vi "ex14-7(withSubVI).vi"() -> ()   [LabVIEW 2014]
panel:
  out "·¸¦ì?65536(­¼ªk)":bool
  out "溢位?65536(除法)":bool
  in  "X":dbl
  in  "Y":dbl
  in  "DIV":bool
  out "X / Y":dbl
  out "X * Y":dbl
  in  "MUX":bool
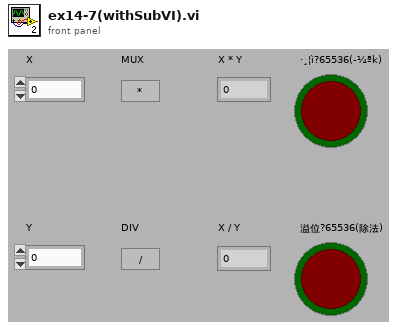
[diagram p1: front panel]
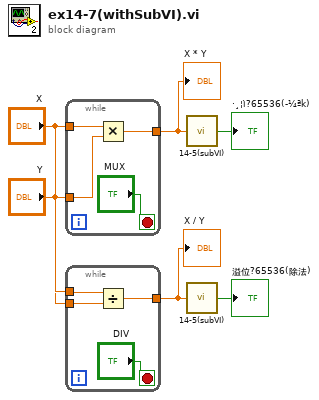
[diagram p0: block diagram]
diagram:
  n1 = while {
    tunnel: [w9] -> w2
    tunnel: "X" -> [w8]
    tunnel: "Y" -> [w7]
    stop <- "MUX" stop-if-true
    n2 = Multiply(x=w8, y=w7) -> (x*y=w9:dbl)
  }
  "X * Y" <- w2
  n3 = while {
    tunnel: [w13] -> w1
    tunnel: "X" -> [w12]
    tunnel: "Y" -> [w11]
    stop <- "DIV" stop-if-true
    n4 = Divide(x=w12, y=w11) -> (x/y=w13:dbl)
  }
  "X / Y" <- w1
  n5 = call "14-5(subVI).vi"("輸入"=w2) -> ("·¸¦ì?65536"=→"·¸¦ì?65536(­¼ªk)":bool)
  n6 = call "14-5(subVI).vi"("輸入"=w1) -> ("·¸¦ì?65536"=→"溢位?65536(除法)":bool)
